vi "Read Theme from Config.vi"(8 "error in":errorcluster) -> (0 "error out":errorcluster, 3 "Theme":bool)   [LabVIEW 2019, in "Panther Dashboard.lvlib"]
uses:
  Panther Dashboard.lvlib
  <vilib>/Utility/config.llb/Read Key (Boolean).vi
  <vilib>/Utility/config.llb/NI_LVConfig.lvlib
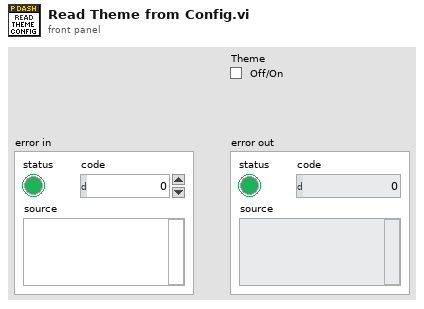
[diagram p1: front panel]
types:
  T1 = typedef "NI_LVConfig.lvlib/Config Data RefNum.ctl" = refnum<k1>
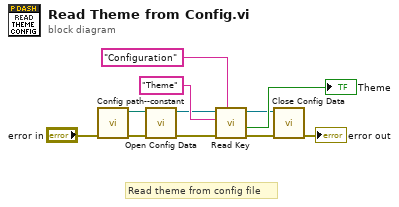
[diagram p0: block diagram]
diagram:
  # "Read theme from config file"
  n1 = call "Config path--constant.vi"("error in (no error)"="error in") -> ("error out"=w8:errorcluster, "Config Path"=w1:path)  [unwired: 9 in]
  n2 = call <vilib>:"Open Config Data.vi"("error in (no error)"=w8, "configuration file path"=w1) -> ("error out"=w11:errorcluster, "refnum"=w3:T1)  [unwired: 7 in, 1 out]
  n3 = call-poly <vilib>:"Read Key.vi"("section"="Configuration", "error in (no error)"=w11, "key"="Theme", "refnum"=w3) -> ("error out"=w10:errorcluster, "value"=→"Theme":bool, "refnum out"=w2:T1)  [unwired: 4 in, 1 out]
  n4 = call <vilib>:"Close Config Data.vi"("error in (no error)"=w10, "refnum"=w2) -> ("error out"=→"error out":errorcluster)  [unwired: 8 in, 1 out]
